vi "Newmark-ExceptionString.vi"(5 "Except NEW":i32, 9 "Except IN":i32) -> (8 "Except OUT":i32)   [LabVIEW 2011]
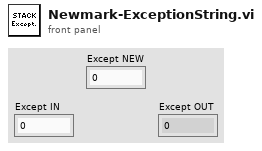
[diagram p1: front panel]
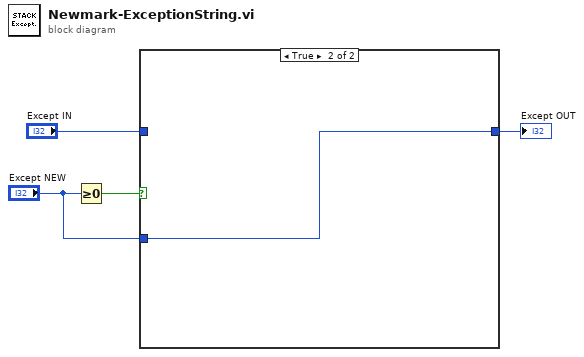
[diagram p0: block diagram]
diagram:
  n1 = Greater Or Equal To 0?(x="Except NEW") -> (x >= 0?=w4:bool)
  n2 = case shown="True" w4 {
    tunnel: "Except IN" -> [w5 _]
    tunnel: [w5 w6] -> w3
    tunnel: "Except NEW" -> [_ w6]
    frame False {
    }
    frame True {
    }
  }
  "Except OUT" <- w3
